vi "launcher fgv.vi"(7 "execution system":T1=enum."standard", 8 "error in":errorcluster, 10 "queue size (1,10000)":i32=1000, 11 "communicator in":refnum<class "communicator.lvclass">) -> (0 "error out":errorcluster, 3 "initialized communicator":refnum<class "communicator.lvclass">)   [LabVIEW 2015, in "communicator manager.lvlib"]
uses:
  communicator manager.lvlib
  communicator/communicator.lvclass
  taskpool/dispatcher/execution system.ctl
  taskpool/dispatcher/pool sizes.ctl
  taskpool/dispatcher/thread pool.lvclass
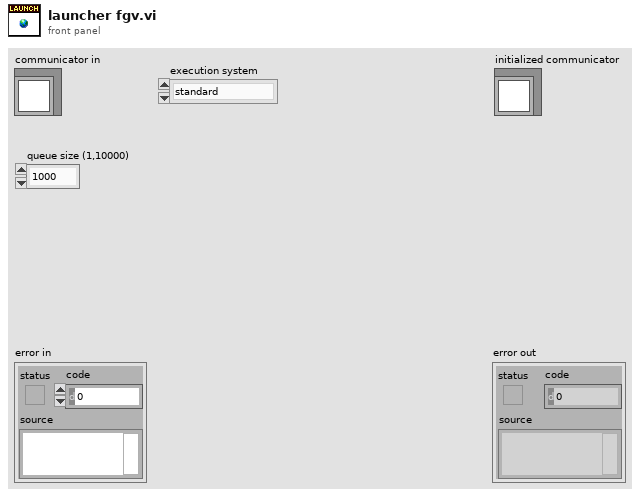
[diagram p1: front panel]
types:
  T1 = typedef "thread pool.lvclass/execution system.ctl" = enum32{"user interface", "standard", "instrument i/o", "data acquisition", "other 1", "other 2"}
  T2 = typedef "thread pool.lvclass/pool sizes.ctl" = cluster{"UI thread":u8, "standard":u8, "instrument I/O":u8, "data acquisition":u8, "other 1":u8, "other 2":u8}
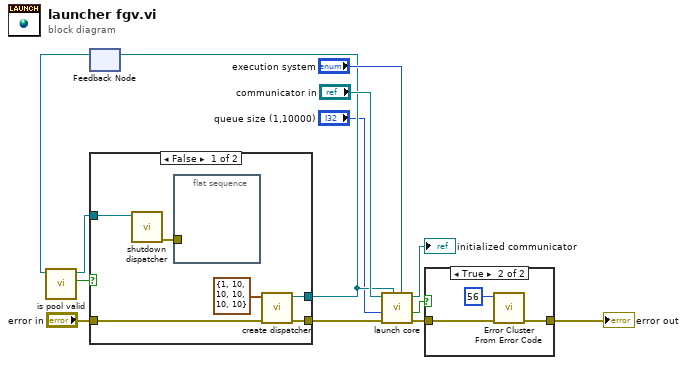
[diagram p0: block diagram]
diagram:
  n1 = feedback #1() -> (w11:refnum<class "thread pool.lvclass">)  [unwired: 1 in]
  n2 = call "is pool valid.vi"("thread pool in"=w11) -> ("valid"=w12:bool, "thread pool out"=w10:refnum<class "thread pool.lvclass">)  [unwired: 9 in]
  n3 = case shown="False" w12 {
    tunnel: [w15 w21] -> w2
    tunnel: w10 -> [w19 w21]
    tunnel: "error in" -> [w17 w20]
    tunnel: [w16 w20] -> w9
    frame False {
      n4 = call "shutdown dispatcher.vi"("thread pool"=w19) -> ("error out"=w18:errorcluster)  [unwired: 10 in]
      n5 = flat-sequence {
        tunnel: w18 -> [_]
        frame #0 {
        }
      }
      n6 = call "create dispatcher.vi"("error in"=w17, "pool sizes (standard=10)"=T2 {"UI thread"=1, "standard"=10, "instrument I/O"=10, "data acquisition"=10, "other 1"=10, "other 2"=10}) -> ("error out"=w16:errorcluster, "dispatcher"=w15:refnum<class "thread pool.lvclass">)  [unwired: 8 in]
    }
    frame True {
    }
  }
  n7 = feedback-in #1(w2) -> ()
  n8 = call "launch core.vi"("execution system"="execution system", "thread pool in"=w2, "error in (no error)"=w9, "queue size"="queue size (1,10000)", "communicator in"="communicator in") -> ("error out"=w5:errorcluster, "timed out?"=w6:bool, "communicator out"=→"initialized communicator":refnum<class "communicator.lvclass">)  [unwired: 4 in]
  n9 = case shown="True" w6 {
    tunnel: w5 -> [w22 w25]
    tunnel: [w22 w24] -> w4
    frame False {
    }
    frame True {
      n10 = call <vilib>:"Error Cluster From Error Code.vi"("error in (no error)"=w25, "error code (0)"=56) -> ("error out"=w24:errorcluster)  [unwired: 7 in]
    }
  }
  "error out" <- w4
